vi "prefiltro.vi"(9 "pk-1":dbl, 10 "pk-2":dbl, 11 "rk-2":dbl) -> (2 "pk":dbl)   [LabVIEW 2019]
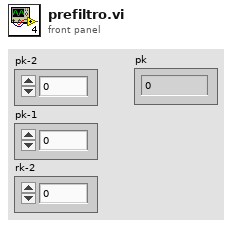
[diagram p1: front panel]
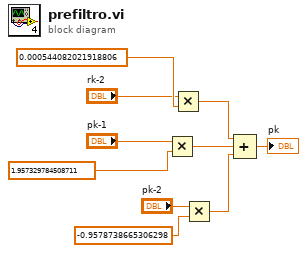
[diagram p0: block diagram]
diagram:
  n1 = Multiply(x="pk-1", y=1.957329784508711) -> (x*y=w8:dbl)
  n2 = Multiply(x="rk-2", y=0.000544082021918806) -> (x*y=w9:dbl)
  n3 = Multiply(x="pk-2", y=-0.9578738665306298) -> (x*y=w7:dbl)
  n4 = Compound Arithmetic op=ADD(w9, w8, w7) -> (→"pk":dbl)
